vi "BRig_Host_dataRunState__entryDelete__updateDataTS.vi"() -> ()   [LabVIEW 2014]
panel:
  in  "output_arrTrials":u16[](array[numeric])
  in  "output_arrTrials_length":i32
  in  "output_arrTrials":bool
  in  "input_row_dataTS":i32
  in  "input_idx":i32[](array[numeric])
  in  "input_dataTS":u16[][](array[numeric])
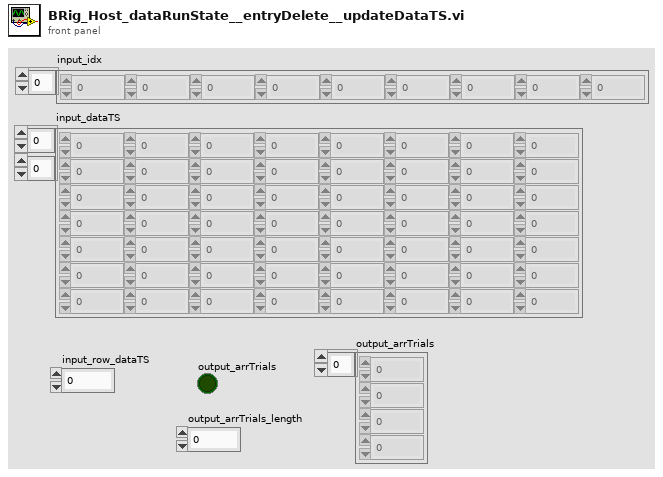
[diagram p1: front panel]
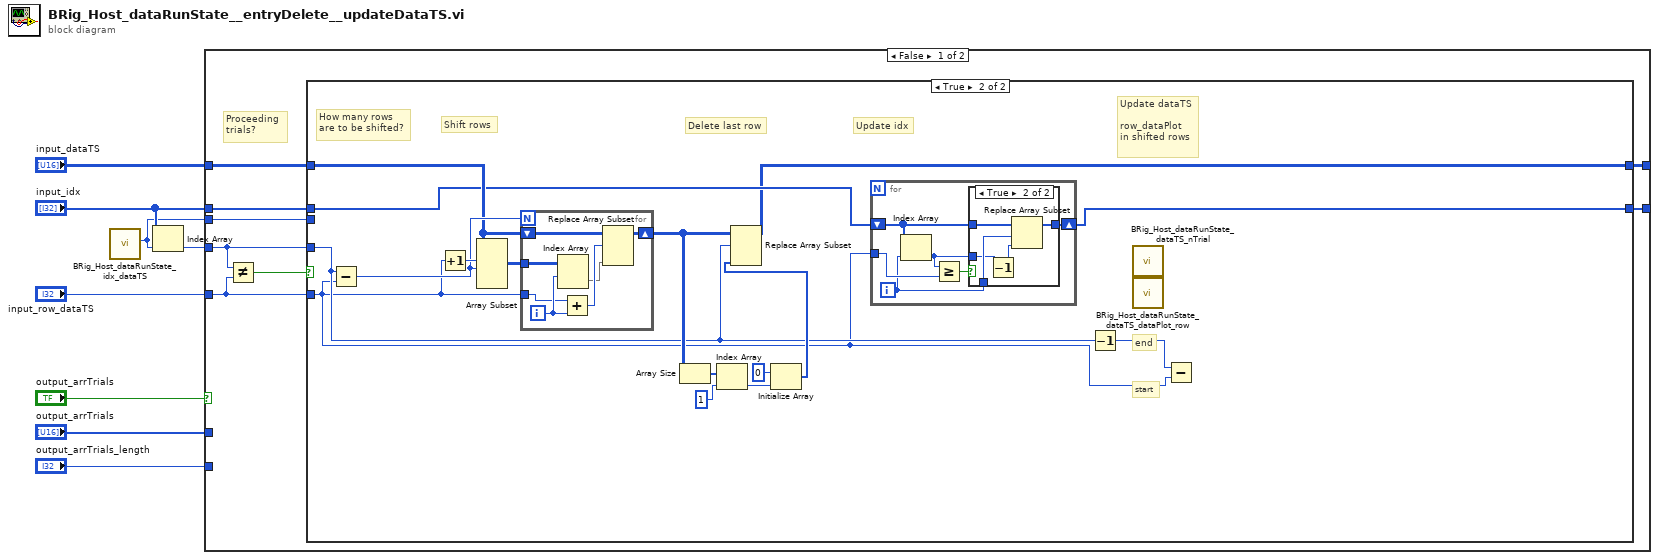
[diagram p0: block diagram]
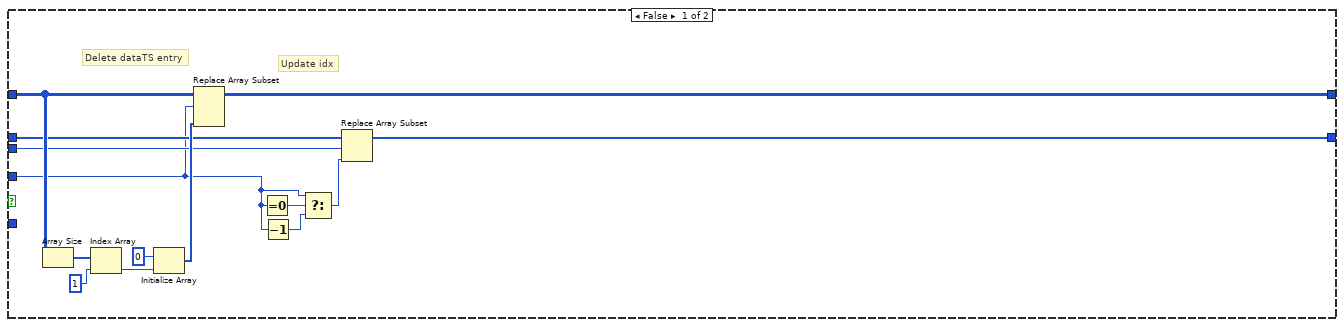
[diagram p2: hidden frame]
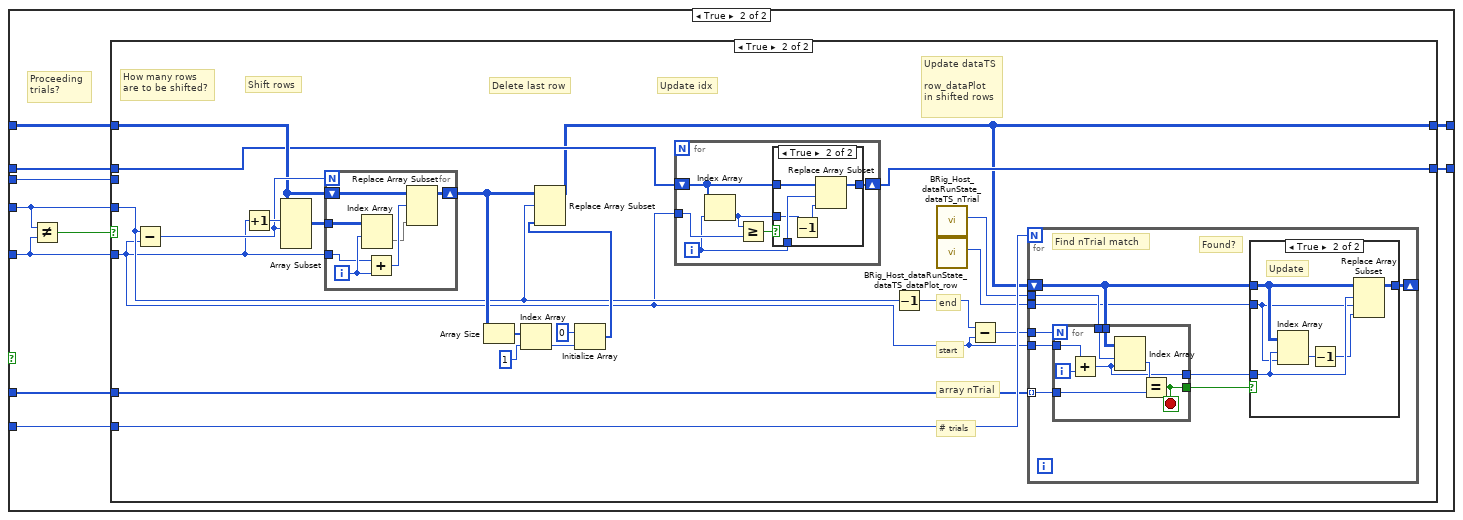
[diagram p4: hidden frame]
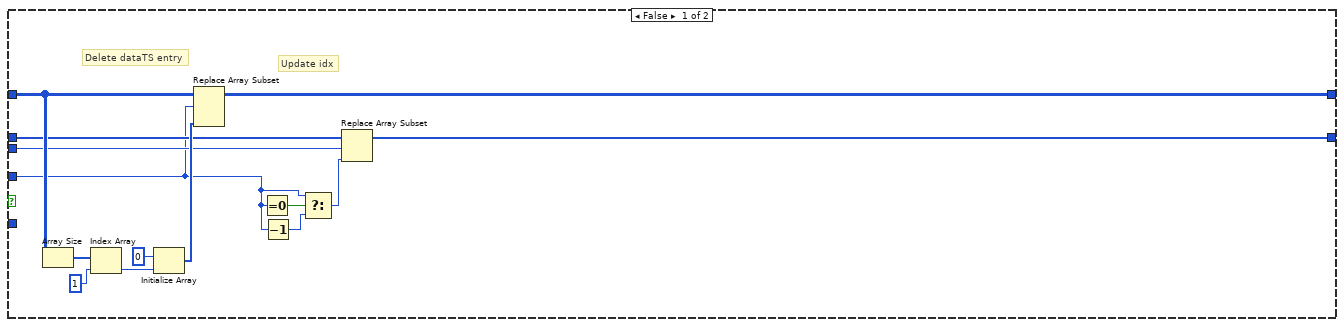
[diagram p5: hidden frame]
diagram:
  n1 = call "BRig_Host_dataRunState_idx_dataTS.vi"() -> ("output_idx_dataTS"=w3:i32)  [unwired: 11 in]
  n2 = Index Array(array="input_idx", index=w3) -> (element=w4:i32)
  n3 = case shown="False" "output_arrTrials" {
    tunnel: "input_idx" -> [w13 w72]
    tunnel: "input_dataTS" -> [w15 w74]
    tunnel: "input_row_dataTS" -> [w9 w68]
    tunnel: w4 -> [w14 w73]
    tunnel: w3 -> [w12 w71]
    tunnel: [w11 w70] -> _
    tunnel: [w10 w69] -> _
    tunnel: "output_arrTrials" -> [_ w67]
    tunnel: "output_arrTrials_length" -> [_ w66]
    frame False {
      # "Proceeding\ntrials?"
      n4 = Not Equal?(x=w14, y=w9) -> (x != y?=w16:bool)
      n5 = case shown="True" w16 {
        tunnel: w15 -> [w30 w44]
        tunnel: w14 -> [w21 w34]
        tunnel: w13 -> [w24 w36]
        tunnel: w12 -> [w23 _]
        tunnel: [w18 w31] -> w11
        tunnel: [w17 w35] -> w10
        tunnel: w9 -> [_ w32]
        frame False {
          # "Update idx"
          # "Delete dataTS entry"
          n6 = Array Size(array=w30) -> (size(s)=w29:i32[])
          n7 = Index Array(array=w29, index=1) -> (element=w27:i32)
          n8 = Initialize Array(u16 0 ("element"), w27) -> (w25:u16[])
          n9 = Replace Array Subset(array=w30, new element=w25, index (row)=w21) -> (w18:u16[][])  [unwired: 1 in]
          n10 = Equal To 0?(x=w21) -> (x = 0?=w22:bool)
          n11 = Decrement(x=w21) -> (x-1=w20:i32)
          n12 = Select(t=w21, s=w22, f=w20) -> (s? t:f=w19:i32)
          n13 = Replace Array Subset(array=w24, new element=w19, index=w23) -> (w17:i32[])
        }
        frame True {
          # "end"
          # "start"
          # "Update dataTS\n\nrow_dataPlot\nin shifted rows"
          # "Update idx"
          # "Delete last row"
          # "Shift rows"
          # "How many rows\nare to be shifted?"
          n14 = Subtract(x=w34, y=w32) -> (x-y=w45:i32)
          n15 = Increment(x=w32) -> (x+1=w46:i32)
          n16 = Array Subset(array=w44, index (row)=w46, length (row)=w45) -> (w43:u16[][])  [unwired: 2 in]
          n17 = for {
            N: w45 -> [_]
            shift-right: [w61] -> w39
            shift-left: w44 -> [w62]
            tunnel: w43 -> [w65]
            tunnel: w32 -> [w63]
            i -> [w64]
            n18 = Index Array(array=w65, index (row)=w64) -> (element=w59:u16[])  [unwired: 1 in]
            n19 = Add(x=w63, y=w64) -> (x+y=w60:i32)
            n20 = Replace Array Subset(array=w62, new element=w59, index (row)=w60) -> (w61:u16[][])  [unwired: 1 in]
          }
          n21 = Array Size(array=w39) -> (size(s)=w42:i32[])
          n22 = Index Array(array=w42, index=1) -> (element=w37:i32)
          n23 = Initialize Array(u16 0 ("element"), w37) -> (w38:u16[])
          n24 = Replace Array Subset(array=w39, new element=w38, index (row)=w34) -> (w31:u16[][])  [unwired: 1 in]
          n25 = for {
            shift-right: [w48] -> w35
            shift-left: w36 -> [w49]
            tunnel: w32 -> [w52]
            i -> [w47]
            n26 = Index Array(array=w49, index=w47) -> (element=w50:i32)
            n27 = Greater Or Equal?(x=w50, y=w52) -> (x >= y?=w51:bool)
            n28 = case shown="True" w51 {
              tunnel: w50 -> [_ w55]
              tunnel: w49 -> [w53 w58]
              tunnel: [w53 w57] -> w48
              tunnel: w47 -> [_ w56]
              frame False {
              }
              frame True {
                n29 = Decrement(x=w55) -> (x-1=w54:i32)
                n30 = Replace Array Subset(array=w58, new element=w54, index=w56) -> (w57:i32[])
              }
            }
          }
          n31 = Decrement(x=w34) -> (x-1=w33:i32)
          n32 = call "BRig_Host_dataRunState_dataTS_nTrial.vi"() -> ()  [unwired: 11 in, 1 out]
          n33 = call "BRig_Host_dataRunState_dataTS_dataPlot_row.vi"() -> ()  [unwired: 11 in, 1 out]
          n34 = Subtract(x=w33, y=w32) -> ()  [unwired: 1 out]
        }
      }
    }
    frame True {
      # "Proceeding\ntrials?"
      n35 = Not Equal?(x=w73, y=w68) -> (x != y?=w75:bool)
      n36 = case shown="True" w75 {
        tunnel: w74 -> [w89 w108]
        tunnel: w73 -> [w80 w98]
        tunnel: w72 -> [w83 w100]
        tunnel: w71 -> [w82 _]
        tunnel: [w77 w92] -> w70
        tunnel: [w76 w99] -> w69
        tunnel: w68 -> [_ w94]
        tunnel: w67 -> [_ w96]
        tunnel: w66 -> [_ w97]
        frame False {
          # "Update idx"
          # "Delete dataTS entry"
          n37 = Array Size(array=w89) -> (size(s)=w88:i32[])
          n38 = Index Array(array=w88, index=1) -> (element=w86:i32)
          n39 = Initialize Array(u16 0 ("element"), w86) -> (w84:u16[])
          n40 = Replace Array Subset(array=w89, new element=w84, index (row)=w80) -> (w77:u16[][])  [unwired: 1 in]
          n41 = Equal To 0?(x=w80) -> (x = 0?=w81:bool)
          n42 = Decrement(x=w80) -> (x-1=w79:i32)
          n43 = Select(t=w80, s=w81, f=w79) -> (s? t:f=w78:i32)
          n44 = Replace Array Subset(array=w83, new element=w78, index=w82) -> (w76:i32[])
        }
        frame True {
          # "array nTrial"
          # "# trials"
          # "end"
          # "start"
          # "Update dataTS\n\nrow_dataPlot\nin shifted rows"
          # "Update idx"
          # "Delete last row"
          # "Shift rows"
          # "How many rows\nare to be shifted?"
          n45 = Subtract(x=w98, y=w94) -> (x-y=w109:i32)
          n46 = Increment(x=w94) -> (x+1=w110:i32)
          n47 = Array Subset(array=w108, index (row)=w110, length (row)=w109) -> (w107:u16[][])  [unwired: 2 in]
          n48 = for {
            N: w109 -> [_]
            shift-right: [w149] -> w103
            shift-left: w108 -> [w150]
            tunnel: w107 -> [w153]
            tunnel: w94 -> [w151]
            i -> [w152]
            n49 = Index Array(array=w153, index (row)=w152) -> (element=w147:u16[])  [unwired: 1 in]
            n50 = Add(x=w151, y=w152) -> (x+y=w148:i32)
            n51 = Replace Array Subset(array=w150, new element=w147, index (row)=w148) -> (w149:u16[][])  [unwired: 1 in]
          }
          n52 = Array Size(array=w103) -> (size(s)=w106:i32[])
          n53 = Index Array(array=w106, index=1) -> (element=w101:i32)
          n54 = Initialize Array(u16 0 ("element"), w101) -> (w102:u16[])
          n55 = Replace Array Subset(array=w103, new element=w102, index (row)=w98) -> (w92:u16[][])  [unwired: 1 in]
          n56 = for {
            shift-right: [w136] -> w99
            shift-left: w100 -> [w137]
            tunnel: w94 -> [w140]
            i -> [w135]
            n57 = Index Array(array=w137, index=w135) -> (element=w138:i32)
            n58 = Greater Or Equal?(x=w138, y=w140) -> (x >= y?=w139:bool)
            n59 = case shown="True" w139 {
              tunnel: w138 -> [_ w143]
              tunnel: w137 -> [w141 w146]
              tunnel: [w141 w145] -> w136
              tunnel: w135 -> [_ w144]
              frame False {
              }
              frame True {
                n60 = Decrement(x=w143) -> (x-1=w142:i32)
                n61 = Replace Array Subset(array=w146, new element=w142, index=w144) -> (w145:i32[])
              }
            }
          }
          n62 = Decrement(x=w98) -> (x-1=w95:i32)
          n63 = call "BRig_Host_dataRunState_dataTS_nTrial.vi"() -> ("output_idx_dataTS_nTrial"=w91:i32)  [unwired: 11 in]
          n64 = call "BRig_Host_dataRunState_dataTS_dataPlot_row.vi"() -> ("output_idx_dataTS_dataPlot_row"=w90:i32)  [unwired: 11 in]
          n65 = Subtract(x=w95, y=w94) -> (x-y=w93:i32)
          n66 = for {
            N: w97 -> [_]
            tunnel: w96 -> [w116] mode=indexing
            tunnel: w94 -> [w118]
            tunnel: w93 -> [w119]
            shift-right: [w112] -> _
            shift-left: w92 -> [w113]
            tunnel: w91 -> [w117]
            tunnel: w90 -> [w111]
            # "Found?"
            # "Find nTrial match"
            n67 = for {
              N: w119 -> [_]
              tunnel: w118 -> [w134]
              tunnel: w113 -> [w132]
              tunnel: w117 -> [w131]
              tunnel: w116 -> [w130]
              tunnel: [w128] -> w115
              tunnel: [w127] -> w114
              i -> [w133]
              stop <- w128 stop-if-true
              n68 = Add(x=w134, y=w133) -> (x+y=w127:i32)
              n69 = Index Array(array=w132, index (row)=w131, index (col)=w127) -> (element=w129:u16)
              n70 = Equal?(x=w129, y=w130) -> (x = y?=w128:bool)
            }
            n71 = case shown="True" w115 {
              tunnel: w114 -> [_ w123]
              tunnel: w113 -> [w120 w125]
              tunnel: [w120 w124] -> w112
              tunnel: w111 -> [_ w122]
              frame False {
              }
              frame True {
                # "Update"
                n72 = Index Array(array=w125, index (row)=w123, index (col)=w122) -> (element=w126:u16)
                n73 = Decrement(x=w126) -> (x-1=w121:u16)
                n74 = Replace Array Subset(array=w125, new element=w121, index (row)=w123, index (col)=w122) -> (w124:u16[][])
              }
            }
          }
        }
      }
    }
  }
